vi "Log.vi"(8 "error in (no error)":errorcluster, 11 "Message Queues in":T1) -> (0 "error out":errorcluster)   [LabVIEW 2020]
uses:
  support/Message Queue/All Message Queues.ctl
  support/Message Queue/Message Cluster.ctl
  Real-Time/controls/Controller Data.ctl
  Real-Time/Control Algorithm/Control Algorithm Data.ctl
  Real-Time/Control Algorithm/Control Algorithm Selection.ctl
  controls/Setpoints.ctl
  support/Message Queue/Message Queue.lvlib
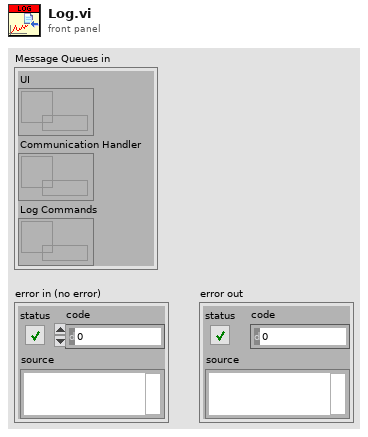
[diagram p1: front panel]
types:
  T1 = typedef "Message Queue.lvlib/All Message Queues.ctl" = cluster{"UI":refnum<queue>, "Communication Handler":refnum<queue>, "Log Commands":refnum<queue>}
  T2 = enum16{"open", "open or create", "create or replace", "create", "open (read-only)"}
  T3 = cluster{"Front panel image path":path, "Log File path":path, "Model path":path}
  T4 = typedef "Controller Data.ctl" = cluster{"Closed Loop Enabled":bool, "Proportional valve 1":dbl, "Proportional valve 2":dbl, "Controller":T5, "Setpoint":T7, "Plant Control Variables":cluster{"Tank 1 Level":dbl, "Tank 2 Level":dbl, "Tank 3 Level":dbl, "Tank 4 Level":dbl, "Pump 1":dbl, "Pump 2":dbl, "Setpoint 1 signal":dbl, "Setpoint 2 signal":dbl}}
  T5 = typedef "Control Algorithm Data.ctl" = cluster{"Control Algorithm":T6, "K":cluster{"A":dbl[][], "B":dbl[][], "C":dbl[][], "D":dbl[][]}, "PI/W1":cluster{"A":dbl[][], "B":dbl[][], "C":dbl[][], "D":dbl[][]}, "W2":cluster{"A":dbl[][], "B":dbl[][], "C":dbl[][], "D":dbl[][]}}
  T6 = typedef "Control Algorithm Selection.ctl" = enum16{"LQG-LTR", "Hinf", "New Controller"}
  T7 = typedef "Setpoints.ctl" = cluster{"Setpoints":cluster{"Setpoint Tank 1":dbl, "Setpoint Tank 2":dbl, "Sin on-off":enum32{"On", "Off"}, "Amplitude Tank 1":dbl, "Amplitude Tank 2":dbl, "Frequency Tank 1":dbl, "Frequency Tank 2":dbl, "Phase Tank 1":dbl, "Phase Tank 2":dbl}, "Disturbance":cluster{"Distubance pump 1":bool, "Amplitude Pump 1":dbl, "Distubance pump 2":bool, "Amplitude Pump 2":dbl}}
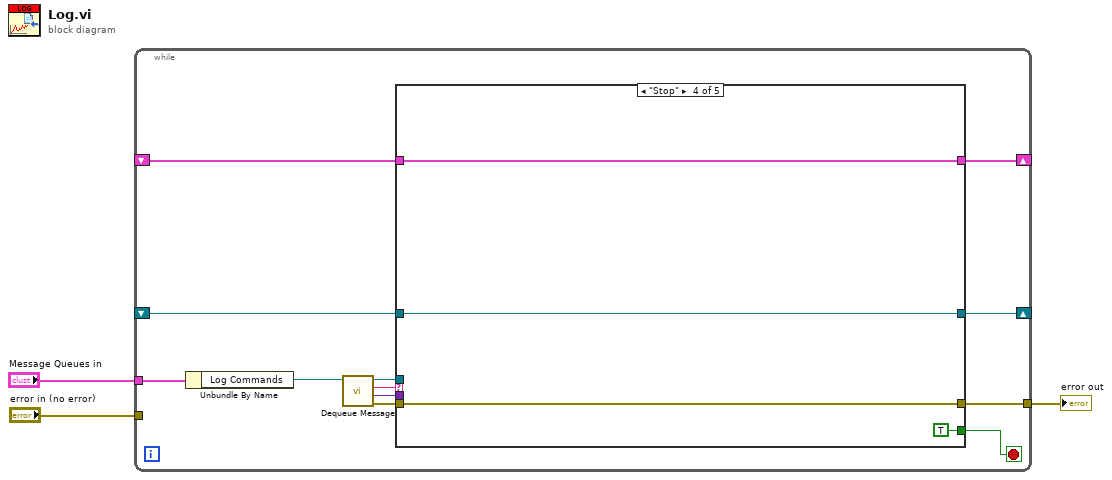
[diagram p0: block diagram]
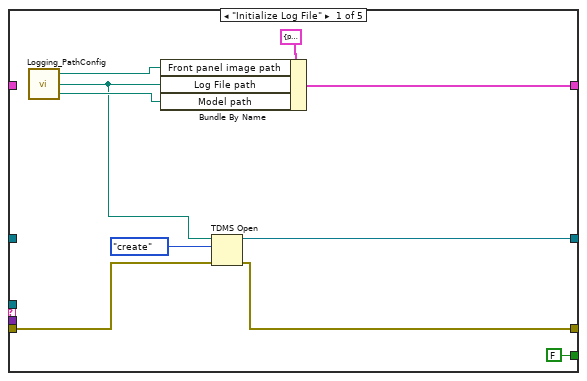
[diagram p2: hidden frame]
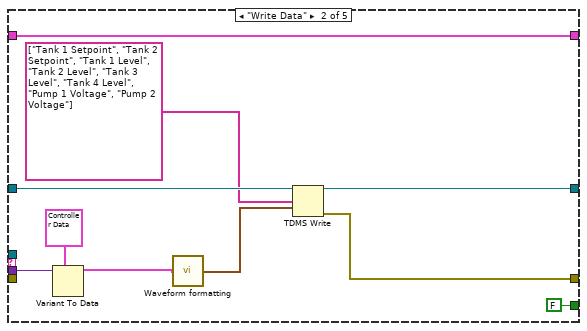
[diagram p3: hidden frame]
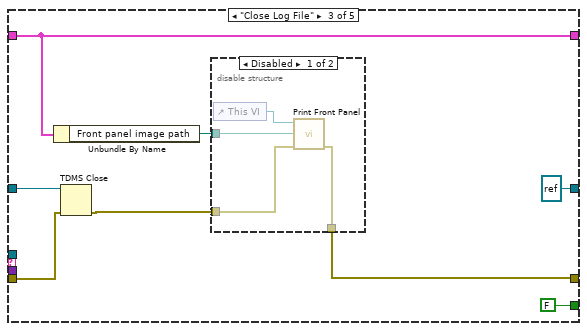
[diagram p4: hidden frame]
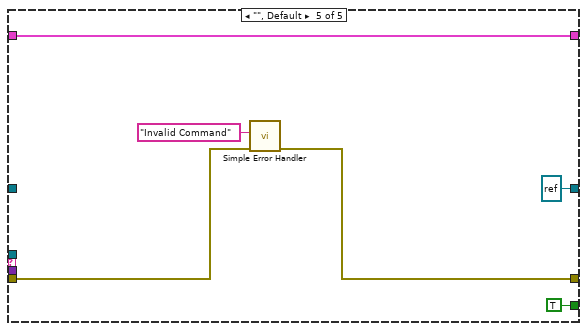
[diagram p6: hidden frame]
diagram:
  n1 = while {
    tunnel: "Message Queues in" -> [w14]
    tunnel: [w10] -> w1
    tunnel: "error in (no error)" -> [_]
    shift-right: [w7] -> _
    shift-left: _ -> [w6]
    shift-right: [w5] -> _
    shift-left: _ -> [w4]
    stop <- w9 stop-if-true
    n2 = Unbundle By Name(w14) -> ("Log Commands"=w13:refnum<queue>)
    n3 = call "Dequeue Message.vi"("Message Queue"=w13) -> ("error out"=w11:errorcluster, "Message Data"=w8:variant, "Message"=w15:string, "dup Message Queue"=w12:refnum<queue>)  [unwired: 7 in]
    n4 = case shown="\"Stop\"" w15 {
      tunnel: w12 -> [_ _ _ _ _]
      tunnel: w11 -> [w19 _ w39 w49 w57]
      tunnel: [w17 w29 w36 w49 w55] -> w10
      tunnel: [FALSE FALSE FALSE TRUE TRUE] -> w9
      tunnel: w8 -> [_ w32 _ _ _]
      tunnel: [w21 w31 w42 w51 w52] -> w7
      tunnel: w6 -> [_ w31 w42 w51 w52]
      tunnel: [w20 w33 refnum<k34> refnum ("tdms file out") w50 refnum<k34> refnum ("tdms file out")] -> w5
      tunnel: w4 -> [_ w34 w40 w50 _]
      frame "Initialize Log File" {
        n5 = call "Logging_PathConfig.vi"() -> ("Front panel image path"=w24:path, "Log File path"=w16:path, "Model path"=w23:path)  [unwired: 5 in]
        n6 = Bundle By Name(cluster=T3 {"Front panel image path"=path "", "Log File path"=path "", "Model path"=path ""}, "Front panel image path"=w24, "Log File path"=w16, "Model path"=w23) -> (w21:T3)
        n7 = TDMS Open(8:w19, 10:T2."create" ("operation (0:open)"), 11:w16) -> (0:w17:errorcluster, 3:w20:refnum<k34>)  [unwired: 4 in]
      }
      frame "Write Data" {
        n8 = Variant To Data(type=T4 {"Closed Loop Enabled"=FALSE, "Proportional valve 1"=0.0, "Proportional valve 2"=0.0, "Controller"={"Control Algorithm"=enum."LQG-LTR", "K"={"A"=[[1.62451, -0.722865, 0.589162, 0.0258055, -0.291247, -0.19871], [0.616764, 0.243215, 0.627021, 0.310989, -0.690401, -0.192347], [-1.01378, 1.19782, 0.595116, 0.307107, -0.873915, -0.221858], [0.460934, 0.301624, 0.892121, 0.145562, -1.07734, -0.276248], [-0.148448, 0.409634, 0.289356, 0.289437, -0.348463, -0.146062], [-0.46568, 0.0291416, 0.0291565, 0.00664228, 0.274253, 0.0367555]], "B"=[[-0.400941, 1.75732], [-0.839249, -0.493575], [-1.18504, -0.379909], [-0.825179, 0.0646258], [0.655259, -0.107787], [0.351957, -0.140832]], "C"=[[0.185781, 0.5585, 1.12711, -0.0910001, -2.59125, -0.578566], [-1.86119, 1.94847, -1.12933, 0.309409, -0.22228, -0.226668]], "D"=[[4.45609, -0.0220273], [-0.0283496, 4.51922]]}, "PI/W1"={"A"=[[-4.94989, 0.0218181, -352.966, 23.8192, -3.10685, -0.000952287], [-0.0218181, -4.904857, 23.4819, -343.472, 0.000977323, -3.58066], [0.0389045, 0.0, -31.6573, 0.0287797, 0.0245405, 0.0], [0.0, 0.0381972, 0.0287797, -31.6573, 0.0, 0.0280468], [0.0, 0.0325383, 0.0240248, -0.0293675, -0.0245405, 0.0], [0.031831, 0.0, -0.0282058, 0.0, 0.0, 0.0]], "B"=[[28.0692, -23.9099], [-23.3912, 28.5852], [31.6468, -0.0287797], [-0.0287797, 31.6468], [-0.0282058, -0.0293675], [0.0282058, -0.0240214]], "C"=[[4.94989, 0.0218181, 314.896, 0.0907351, 3.10685, 0.000952287], [10.0218181, 4.90457, -0.0906726, 314.884, -0.000977323, 3.58066]], "D"=[[0.0, 0.0], [0.0, 0.0]]}, "W2"={"A"=[[-4.94989, 0.0218181, -352.966, 23.8192, -3.10685, -0.000952287], [-0.0218181, -4.904857, 23.4819, -343.472, 0.000977323, -3.58066], [0.0389045, 0.0, -31.6573, 0.0287797, 0.0245405, 0.0], [0.0, 0.0381972, 0.0287797, -31.6573, 0.0, 0.0280468], [0.0, 0.0325383, 0.0240248, -0.0293675, -0.0245405, 0.0], [0.031831, 0.0, -0.0282058, 0.0, 0.0, 0.0]], "B"=[[28.0692, -23.9099], [-23.3912, 28.5852], [31.6468, -0.0287797], [-0.0287797, 31.6468], [-0.0282058, -0.0293675], [0.0282058, -0.0240214]], "C"=[[4.94989, 0.0218181, 314.896, 0.0907351, 3.10685, 0.000952287], [10.0218181, 4.90457, -0.0906726, 314.884, -0.000977323, 3.58066]], "D"=[[0.0, 0.0], [0.0, 0.0]]}}, "Setpoint"={"Setpoints"={"Setpoint Tank 1"=0.0, "Setpoint Tank 2"=0.0, "Sin on-off"=enum."On", "Amplitude Tank 1"=0.0, "Amplitude Tank 2"=0.0, "Frequency Tank 1"=0.0, "Frequency Tank 2"=0.0, "Phase Tank 1"=0.0, "Phase Tank 2"=0.0}, "Disturbance"={"Distubance pump 1"=FALSE, "Amplitude Pump 1"=0.0, "Distubance pump 2"=FALSE, "Amplitude Pump 2"=0.0}}, "Plant Control Variables"={"Tank 1 Level"=0.0, "Tank 2 Level"=0.0, "Tank 3 Level"=0.0, "Tank 4 Level"=0.0, "Pump 1"=0.0, "Pump 2"=0.0, "Setpoint 1 signal"=0.0, "Setpoint 2 signal"=0.0}} ("Cluster"), Variant=w32) -> (data=w28:T4)  [unwired: 1 in, 1 out]
        n9 = call "Waveform formatting.vi"("Cluster"=w28) -> ("Tank Levels"=w27:waveform(dbl)[])
        n10 = TDMS Write(0:w34, 7:string[] ["Tank 1 Setpoint", "Tank 2 Setpoint", "Tank 1 Level", "Tank 2 Level", "Tank 3 Level", "Tank 4 Level", "Pump 1 Voltage", "Pump 2 Voltage"], 9:w27) -> (4:w33:refnum<k34>, 15:w29:errorcluster)  [unwired: 3 in, 2 out]
      }
      frame "Close Log File" {
        n11 = Unbundle By Name(w42) -> ("Front panel image path"=w41:path)
        n12 = TDMS Close(8:w39, 11:w40) -> (0:w38:errorcluster)  [unwired: 1 out]
        n13 = disable-structure shown="Disabled" {
          disable-tunnel: w41 -> [w46 _]
          disable-tunnel: w38 -> [w45 _]
          disable-tunnel: [w44 _] -> w36
          frame Disabled {
            n14 = control-ref of="This VI"() -> (w47:refnum<vi>)
            n15 = call "Print Front Panel.vi"("error in (no error)"=w45, "Front panel image path"=w46, "VI in"=w47) -> ("error out"=w44:errorcluster)  [unwired: 8 in]
          }
          frame Enabled {
          }
        }
      }
      frame "Stop" {
      }
      frame "", Default {
        n16 = call <vilib>:"Simple Error Handler.vi"("error source (\" \")"="Invalid Command" ("error source (\" \")"), "error in (no error)"=w57) -> ("error out"=w55:errorcluster)  [unwired: 3 in, 4 out]
      }
    }
  }
  "error out" <- w1
